vi "KE622x -- 2182 -A Get NPLCs.vi"(0 "622x Resource In":refnum<visa-resource-name>, 1 "Check For SCPI Errors? (T)":bool=TRUE, 11 "error in (no error)":errorcluster) -> (4 "622x Resource Out (dupl)":refnum<visa-resource-name>, 8 "2182 -A NPLCs":T1 min=1 max=60, 15 "error out":errorcluster)   [LabVIEW 2019, in "Keithley 622x.lvlib"]
uses:
  Keithley 622x.lvlib
  Typedefs/KE2182 -- NPLCs.ctl
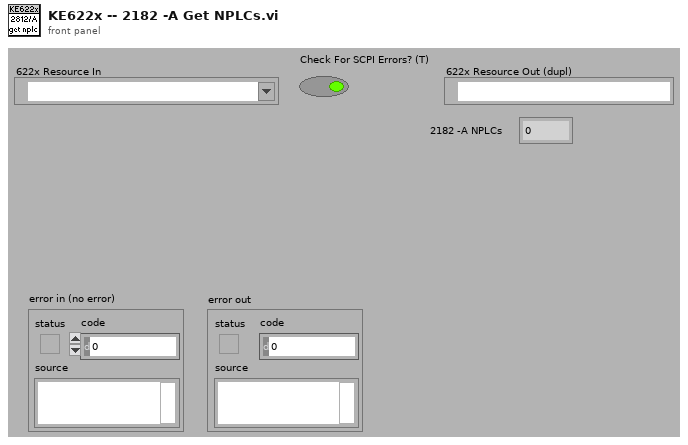
[diagram p1: front panel]
types:
  T1 = typedef "Keithley 622x.lvlib/KE2182 -- NPLCs.ctl" = u32
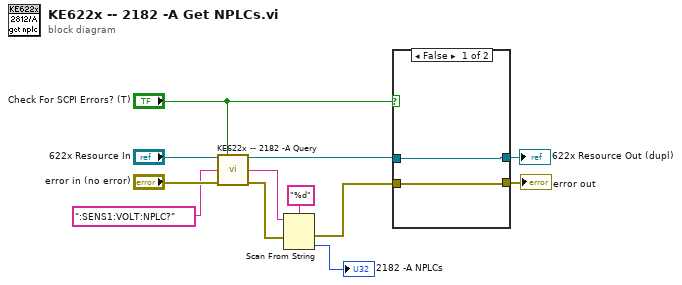
[diagram p0: block diagram]
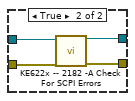
[diagram p2: hidden frame]
diagram:
  n1 = call "KE622x -- 2182 -A Query.vi"("622x Resource In"="622x Resource In", "Check For SCPI Errors? (T)"="Check For SCPI Errors? (T)", "2182-A Write String"=":SENS1:VOLT:NPLC?", "error in (no error)"="error in (no error)") -> ("622x Resource Out (dupl)"=w6:refnum<visa-resource-name>, "2182-A Reponse String"=w7:string, "error out"=w9:errorcluster)  [unwired: 9 in]
  n2 = Scan From String(format string="%d", input string=w7, error in=w9) -> (error out=w5:errorcluster, output 1=→"2182 -A NPLCs":T1)  [unwired: 2 in, 2 out]
  n3 = case shown="False" "Check For SCPI Errors? (T)" {
    tunnel: w6 -> [w14 w18]
    tunnel: w5 -> [w13 w17]
    tunnel: [w14 w16] -> w3
    tunnel: [w13 w15] -> w2
    frame False {
    }
    frame True {
      n4 = call "KE622x -- 2182 -A Check For SCPI Errors.vi"("VISA Resource In"=w18, "error in (no error)"=w17) -> ("VISA Resource Out (dupl)"=w16:refnum<visa-resource-name>, "error out"=w15:errorcluster)  [unwired: 10 in, 2 out]
    }
  }
  "622x Resource Out (dupl)" <- w3
  "error out" <- w2
